vi "TPNT_DeleteDeviceTP.vi"(8 "error in (no error)":errorcluster, 10 "TP name":string, 11 "Object Refnum In":T1) -> (0 "error out":errorcluster, 3 "Data Refnum out":T1)   [LabVIEW 2016]
uses:
  TPNT_Refnum.ctl
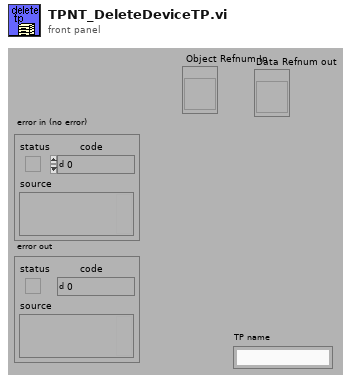
[diagram p1: front panel]
types:
  T1 = typedef "TPNT_Refnum.ctl" = refnum<vi>
  T2 = typedef "TPNT_DeviceTPs.ctl" = cluster{"device":string, "devupdate":dbl, "next_update":u32, "devinterface":string, "TPs":T3[], "Alarms":bool, "monitor":bool, "log sep":string}
  T3 = typedef "TPNT_TP.ctl" = cluster{"name":string, "type":string, "algor":string[], "update_rate":sgl, "Limits":T4, "Samples":T5, "next_update":u32, "Status":string, "monitor":bool, "error":bool, "Log":T6, "permissions":string, "ID":string}
  T4 = typedef "TPNT_Limits.ctl" = cluster{"Alarm Type":string, "Lower ":dbl, "Upper":dbl, "Nominal":dbl, "outrange":bool, "Check":bool, "latch":bool, "level":string}
  T5 = typedef "TPNT_Samples.ctl" = cluster{"samples":i32, "counter":i32, "Values":dbl[], "Current Value":string, "filter":string, "precision":u8}
  T6 = typedef "TPNT_Log.ctl" = cluster{"log":bool, "file":path, "type":string, "format":string, "updaterate":dbl, "nex_update":u32, "mode":string}
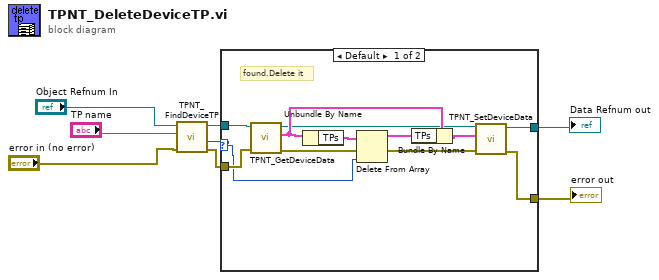
[diagram p0: block diagram]
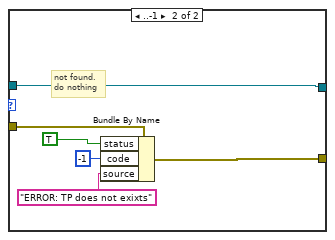
[diagram p2: hidden frame]
diagram:
  n1 = call "TPNT_FindDeviceTP.vi"("error in (no error)"="error in (no error)", "TP name"="TP name", "Object Refnum In"="Object Refnum In") -> ("error out"=w5:errorcluster, "index"=w8:i32, "Data Refnum out"=w3:T1)  [unwired: 1 in, 5 out]
  n2 = case shown="Default" w8 {
    selector: w8 -> [w10 _]
    tunnel: w5 -> [w18 w24]
    tunnel: [w11 w21] -> w4
    tunnel: w3 -> [w19 w20]
    tunnel: [w9 w20] -> w1
    frame Default {
      # "found.Delete it"
      n3 = call "TPNT_GetDeviceData.vi"("error in (no error)"=w18, "Object Refnum In"=w19) -> ("error out"=w12:errorcluster, "Object Data Out"=w15:T2, "Data Refnum out"=w14:T1)  [unwired: 7 out]
      n4 = Unbundle By Name(w15) -> ("TPs"=w17:T3[])
      n5 = Delete From Array(array=w17, index=w10) -> (array with subset deleted=w16:T3[])  [unwired: 1 in, 1 out]
      n6 = Bundle By Name(cluster=w15, "TPs"=w16) -> (w13:T2)
      n7 = call "TPNT_SetDeviceData.vi"("error in (no error)"=w12, "Object Data In"=w13, "Object Refnum In"=w14) -> ("error out"=w11:errorcluster, "Data Refnum out"=w9:T1)  [unwired: 7 out]
    }
    frame ..-1 {
      # "not found.\ndo nothing"
      n8 = Bundle By Name(cluster=w24, "status"=TRUE, "code"=-1, "source"="ERROR: TP does not exixts") -> (w21:errorcluster)
    }
  }
  "Data Refnum out" <- w1
  "error out" <- w4
